vi "ControlForceIdle (1).vi"(10 "Enabled":bool, 11 "Phase in":T1=enum."Idle") -> (3 "Phase out":T1=enum."Idle")   [LabVIEW 2017]
uses:
  StateList.ctl
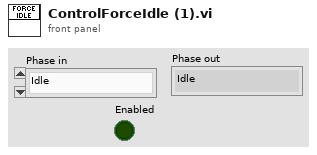
[diagram p1: front panel]
types:
  T1 = typedef "StateList.ctl" = enum16{"Fault", "Idle", "Ready", "Pushing", "Coast", "Braking"}
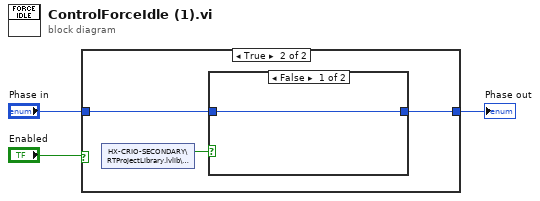
[diagram p0: block diagram]
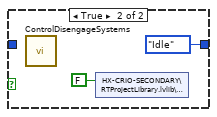
[diagram p3: hidden frame]
diagram:
  n1 = case shown="True" "Enabled" {
    tunnel: [w4 w7] -> w3
    tunnel: "Phase in" -> [w4 w6]
    frame False {
    }
    frame True {
      n2 = shared-variable "HX-CRIO-SECONDARY\\RTProjectLibrary.lvlib\\ForceIdle"() -> (w5:bool)  [unwired: 1 in, 1 out]
      n3 = case shown="False" w5 {
        tunnel: [w8 StateList."Idle" ("Start Phase")] -> w7
        tunnel: w6 -> [w8 _]
        frame False {
        }
        frame True {
          n4 = call "ControlDisengageSystems.vi"() -> ()  [unwired: 12 in]
          n5 = shared-variable "HX-CRIO-SECONDARY\\RTProjectLibrary.lvlib\\ForceIdle"(FALSE ("ForceIdle")) -> ()  [unwired: 1 in, 1 out]
        }
      }
    }
  }
  "Phase out" <- w3
